vi "M14_Turret_Hardware_Loop.vi"   [LabVIEW 2019]
uses:
  Subsystems/Drive/Drive_Globals.vi
  <vilib>/Rock Robotics/WPI/ThirdParty/Phoenix-LabVIEW/Motor Controller/Controls/CTRE_Phoenix_MotorControl_ControlMode.ctl
  M14 Turret_Hardware_Globals.vi
types:
  T1 = typedef "WPI_MotorControlDeviceRef.ctl" = cluster{"DeviceStatus":errorcluster, "Type":T2, "PWM":cluster{"PWM Channel":T3, "DeadBand":T4}, "CAN":cluster{"Device Number":u8, "SetOutput VI Ref":variant, "GetOutput VI Ref":variant, "Enable VI Ref":variant, "Disable VI Ref":variant, "Data":variant}, "Invert":bool, "DIO PWM":cluster{"PWM \"Enable\" Channel":T3, "DIOChannel":T5, "PWM Rate":dbl}}
  T2 = typedef "WPI_MotorControlType.ctl" = enum16{"PWM", "CAN", "DIO PWM"}
  T3 = typedef "FPGA_DIOPWMChannel.ctl" = enum8{"PWM 0", "PWM 1", "PWM 2", "PWM 3", "PWM 4", "PWM 5", "PWM 6", "PWM 7", "PWM 8", "PWM 9", "PWM MXP 0", "PWM MXP 1", "PWM MXP 2", "PWM MXP 3", "PWM MXP 4", "PWM MXP 5", "PWM MXP 6", "PWM MXP 7", "PWM MXP 8", "PWM MXP 9", "Invalid"}
  T4 = typedef "WPI_PWMDeadband.ctl" = cluster{"Name":string, "maxPositivePwm":i32, "minPositivePwm":i32, "centerPwm":i32, "maxNegativePwm":i32, "minNegativePwm":i32, "angularRange":u16}
  T5 = typedef "FPGA_DIOChannel.ctl" = enum8{"DIO 0", "DIO 1", "DIO 2", "DIO 3", "DIO 4", "DIO 5", "DIO 6", "DIO 7", "DIO 8", "DIO 9", "DIO MXP 0", "DIO MXP 1", "DIO MXP 2", "DIO MXP 3", "DIO MXP 4", "DIO MXP 5", "DIO MXP 6", "DIO MXP 7", "DIO MXP 8", "DIO MXP 9", "DIO MXP 10", "DIO MXP 11", "DIO MXP 12", "DIO MXP 13", "DIO MXP 14", "DIO MXP 15", "SPI Port CS1", "SPI Port CS2", "SPI Port CS3", "SPI Port MISO", "SPI Port MOSI", "Invalid"}
  T6 = typedef "Basic_Motor_Modes.ctl" = enum16{"Percent_Voltage", "Speed_Control", "Position_Control", "Current"}
  T7 = typedef "CTRE_Phoenix_MotorControl_ControlMode.ctl" = u16
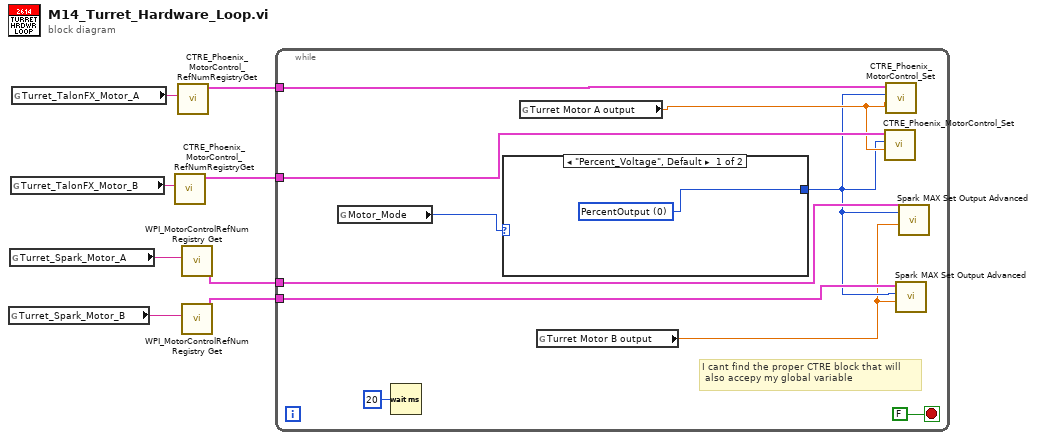
[diagram p0: block diagram]
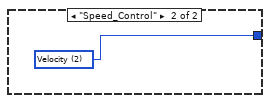
[diagram p2: hidden frame]
diagram:
  n1 = global read "M14 Turret_Hardware_Globals.vi" "Turret_Spark_Motor_B"() -> (w2:string)
  n2 = global read "M14 Turret_Hardware_Globals.vi" "Turret_Spark_Motor_A"() -> (w3:string)
  n3 = global read "M14 Turret_Hardware_Globals.vi" "Turret_TalonFX_Motor_B"() -> (w5:string)
  n4 = global read "M14 Turret_Hardware_Globals.vi" "Turret_TalonFX_Motor_A"() -> (w6:string)
  n5 = call <vilib>:"CTRE_Phoenix_MotorControl_RefNumRegistryGet.vi"("refnum name"=w5) -> ("PhoenixMotorControlDevRef"=w7:T1)  [unwired: 9 in, 1 out]
  n6 = call <vilib>:"CTRE_Phoenix_MotorControl_RefNumRegistryGet.vi"("refnum name"=w6) -> ("PhoenixMotorControlDevRef"=w8:T1)  [unwired: 9 in, 1 out]
  n7 = call <vilib>:"WPI_MotorControlRefNum Registry Get.vi"("refnum name"=w3) -> ("MotorControlDevRef"=w4:T1)  [unwired: 9 in, 1 out]
  n8 = call <vilib>:"WPI_MotorControlRefNum Registry Get.vi"("refnum name"=w2) -> ("MotorControlDevRef"=w1:T1)  [unwired: 9 in, 1 out]
  n9 = while {
    tunnel: w8 -> [w15]
    tunnel: w7 -> [w14]
    tunnel: w4 -> [w12]
    tunnel: w1 -> [w11]
    stop <- FALSE stop-if-true
    # "I cant find the proper CTRE block that will\n also accepy my global variable"
    n10 = global read "Drive_Globals.vi" "Motor_Mode"() -> (w16:T6)
    n11 = Wait (ms)(milliseconds to wait=u32 20) -> ()  [unwired: 1 out]
    n12 = case shown="\"Percent_Voltage\", Default" w16 {
      tunnel: [w19 w20] -> w10
      frame "Percent_Voltage", Default {
        w19 = T7 0 items=["PercentOutput"=0, "Position"=1, "Velocity"=2, "Current"=3, "Follower"=5, "MotionProfile"=6, "MotionMagic"=7, "MotionProfileArc"=10, "Disabled"=15] ("Control Mode")
      }
      frame "Speed_Control" {
        w20 = T7 2 items=["PercentOutput"=0, "Position"=1, "Velocity"=2, "Current"=3, "Follower"=5, "MotionProfile"=6, "MotionMagic"=7, "MotionProfileArc"=10, "Disabled"=15] ("Control Mode")
      }
    }
    n13 = global read "M14 Turret_Hardware_Globals.vi" "Turret Motor A output"() -> (w13:dbl)
    n14 = global read "M14 Turret_Hardware_Globals.vi" "Turret Motor B output"() -> (w9:dbl)
    n15 = call <vilib>:"CTRE_Phoenix_MotorControl_Set.vi"("Output"=w13, "Control Mode"=w10, "PhoenixMotorControlDevRef"=w14) -> ()  [unwired: 7 in, 2 out]
    n16 = call <vilib>:"CTRE_Phoenix_MotorControl_Set.vi"("Output"=w13, "Control Mode"=w10, "PhoenixMotorControlDevRef"=w15) -> ()  [unwired: 7 in, 2 out]
    n17 = call <vilib>:"Spark MAX Set Output Advanced.vi"("Control Mode"=w9, "Setpoint"=w10, "MotorControlDevRef"=w11) -> ()  [unwired: 7 in, 2 out]
    n18 = call <vilib>:"Spark MAX Set Output Advanced.vi"("Control Mode"=w9, "Setpoint"=w10, "MotorControlDevRef"=w12) -> ()  [unwired: 7 in, 2 out]
  }
